vi "Quad Ctr - subVI.vi"(1 "Quadrature Encoder Type":T1(ring), 2 "Steps per Revolution":dbl, 3 "16 bit Position 4":i32) -> (0 "Position (Degrees)":dbl)   [LabVIEW 8.6]
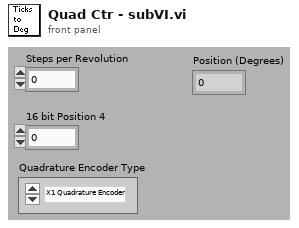
[diagram p1: front panel]
types:
  T1 = enum16{"X1 Quadrature Encoder", "X2 Quadrature Encoder", "X4 Quadrature Encoder"}
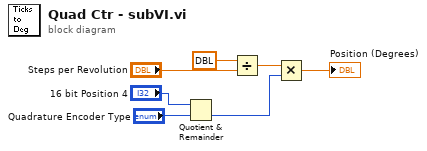
[diagram p0: block diagram]
diagram:
  n1 = Quotient & Remainder(x="16 bit Position 4", y="Quadrature Encoder Type") -> (floor(x/y)=w2:i32)  [unwired: 1 out]
  n2 = Divide(x=dbl ?, y="Steps per Revolution") -> (x/y=w5:dbl)
  n3 = Multiply(x=w5, y=w2) -> (x*y=→"Position (Degrees)":dbl)
